vi "SendChargingCAN.vi"(8 "error in (no error)":errorcluster, 11 "interface object in":refnum<k20>) -> (0 "error out":errorcluster, 3 "interface object out":refnum<k20>)   [LabVIEW 2014]
uses:
  <vilib>/RioEmbeddedCAN/RioEmbeddedCAN.llb/CANFrameControl.ctl
  <vilib>/RioEmbeddedCAN/RioEmbeddedCAN.llb/CANWaitTransmitComplete.vi
  Global Data.vi
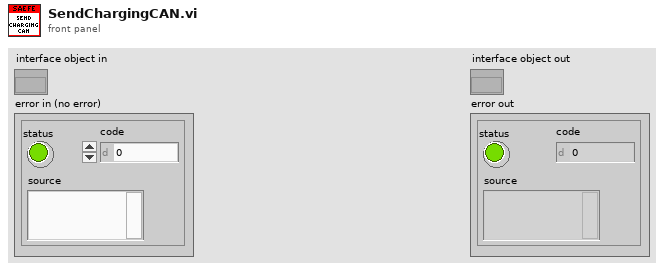
[diagram p1: front panel]
types:
  T1 = typedef "CANFrameControl.ctl" = cluster{"identifier":u32, "extended?":bool, "type":u8, "payload":u8[]}
  T2 = typedef "BMS Telemetry.ctl" = cluster{"bBMSIgnition":bool, "bBMSChargerMains":bool, "bBMSFastCharge":bool, "bBMSChargerEnabled":bool, "eBMSCarState":enum16{"Off", "On, Not Charging", "Charging", "Charging Finished", "Charging Error"}, "eBMSChargingState":enum16{"Disconnected", "Pre-charging", "Main Charging", "Balancing", "Charging Finished OK", "Charging Error"}, "tBMSChargeStage":u16, "eBMSLastChargeError":enum16{"No Error", "No Cell Communication", "No Cell Communication - Non CAN Charger", "Maximum charging stage duration expired", "Cell Communication Lost during Charge", "Cannot set balancing voltage", "Cell temps too high", "No Comms so can't determine temp", "# of Cells Mismatch", "Cells Overvoltage", "Cell Protection Event occured."}, "NBMSNumCells":u8, "bBMSUnderVProtection":bool, "bBMSOverVProtection":bool, "bBMSOverTProtection":bool, "bBMSLeakageProtection":bool, "bBMSNoCellCommsError":bool, "bBMSLowVReduction":bool, "bBMSHighTReduction":bool, "VCellMin":dbl, "VCellMax":dbl, "VCellMean":dbl, "VTotal":dbl, "TCellMin":dbl, "TCellMax":dbl, "TCellMean":dbl, "VCells":cluster{"[51]":dbl, "[52]":dbl, "[53]":dbl, "[54]":dbl, "[55]":dbl, "[56]":dbl, "[57]":dbl, "[58]":dbl, "[59]":dbl, "[60]":dbl, "[61]":dbl, "[62]":dbl, "[63]":dbl, "[64]":dbl, "[65]":dbl, "[66]":dbl, "[67]":dbl, "[34]":dbl, "[35]":dbl, "[36]":dbl, "[37]":dbl, "[38]":dbl, "[39]":dbl, "[40]":dbl, "[41]":dbl, "[42]":dbl, "[43]":dbl, "[44]":dbl, "[45]":dbl, "[46]":dbl, "[47]":dbl, "[48]":dbl, "[49]":dbl, "[50]":dbl, "[17]":dbl, "[18]":dbl, "[19]":dbl, "[20]":dbl, "[21]":dbl, "[22]":dbl, "[23]":dbl, "[24]":dbl, "[25]":dbl, "[26]":dbl, "[27]":dbl, "[28]":dbl, "[29]":dbl, "[30]":dbl, "[31]":dbl, "[32]":dbl, "[33]":dbl, "[0]":dbl, "[1]":dbl, "[2]":dbl, "[3]":dbl, "[4]":dbl, "[5]":dbl, "[6]":dbl, "[7]":dbl, "[8]":dbl, "[9]":dbl, "[10]":dbl, "[11]":dbl, "[12]":dbl, "[13]":dbl, "[14]":dbl, "[15]":dbl, "[16]":dbl}, "TCells":cluster{"[55]":dbl, "[56]":dbl, "[57]":dbl, "[58]":dbl, "[59]":dbl, "[60]":dbl, "[61]":dbl, "[62]":dbl, "[63]":dbl, "[64]":dbl, "[65]":dbl, "[66]":dbl, "[67]":dbl, "[68]":dbl, "[69]":dbl, "[70]":dbl, "[17]":dbl, "[38]":dbl, "[39]":dbl, "[40]":dbl, "[41]":dbl, "[42]":dbl, "[43]":dbl, "[44]":dbl, "[45]":dbl, "[46]":dbl, "[47]":dbl, "[48]":dbl, "[49]":dbl, "[50]":dbl, "[51]":dbl, "[52]":dbl, "[53]":dbl, "[54]":dbl, "[21]":dbl, "[22]":dbl, "[23]":dbl, "[24]":dbl, "[25]":dbl, "[26]":dbl, "[27]":dbl, "[28]":dbl, "[29]":dbl, "[30]":dbl, "[31]":dbl, "[32]":dbl, "[33]":dbl, "[34]":dbl, "[35]":dbl, "[36]":dbl, "[37]":dbl, "[0]":dbl, "[1]":dbl, "[2]":dbl, "[3]":dbl, "[4]":dbl, "[5]":dbl, "[6]":dbl, "[7]":dbl, "[8]":dbl, "[9]":dbl, "[10]":dbl, "[11]":dbl, "[12]":dbl, "[13]":dbl, "[14]":dbl, "[15]":dbl, "[16]":dbl}, "bChargerConnected":bool, "VChargerSetpoint":dbl, "IChargerSetpoint":dbl, "VChargerActual":dbl, "IChargerActual":dbl, "BCells":cluster{"[51]":dbl, "[52]":dbl, "[53]":dbl, "[54]":dbl, "[55]":dbl, "[56]":dbl, "[57]":dbl, "[58]":dbl, "[59]":dbl, "[60]":dbl, "[61]":dbl, "[62]":dbl, "[63]":dbl, "[64]":dbl, "[65]":dbl, "[66]":dbl, "[67]":dbl, "[34]":dbl, "[35]":dbl, "[36]":dbl, "[37]":dbl, "[38]":dbl, "[39]":dbl, "[40]":dbl, "[41]":dbl, "[42]":dbl, "[43]":dbl, "[44]":dbl, "[45]":dbl, "[46]":dbl, "[47]":dbl, "[48]":dbl, "[49]":dbl, "[50]":dbl, "[17]":dbl, "[18]":dbl, "[19]":dbl, "[20]":dbl, "[21]":dbl, "[22]":dbl, "[23]":dbl, "[24]":dbl, "[25]":dbl, "[26]":dbl, "[27]":dbl, "[28]":dbl, "[29]":dbl, "[30]":dbl, "[31]":dbl, "[32]":dbl, "[33]":dbl, "[0]":dbl, "[1]":dbl, "[2]":dbl, "[3]":dbl, "[4]":dbl, "[5]":dbl, "[6]":dbl, "[7]":dbl, "[8]":dbl, "[9]":dbl, "[10]":dbl, "[11]":dbl, "[12]":dbl, "[13]":dbl, "[14]":dbl, "[15]":dbl, "[16]":dbl}}
  T3 = enum16{"Disconnected", "Pre-charging", "Main Charging", "Balancing", "Charging Finished OK", "Charging Error"}
  T4 = enum16{"No Error", "No Cell Communication", "No Cell Communication - Non CAN Charger", "Maximum charging stage duration expired", "Cell Communication Lost during Charge", "Cannot set balancing voltage", "Cell temps too high", "No Comms so can't determine temp", "# of Cells Mismatch", "Cells Overvoltage", "Cell Protection Event occured."}
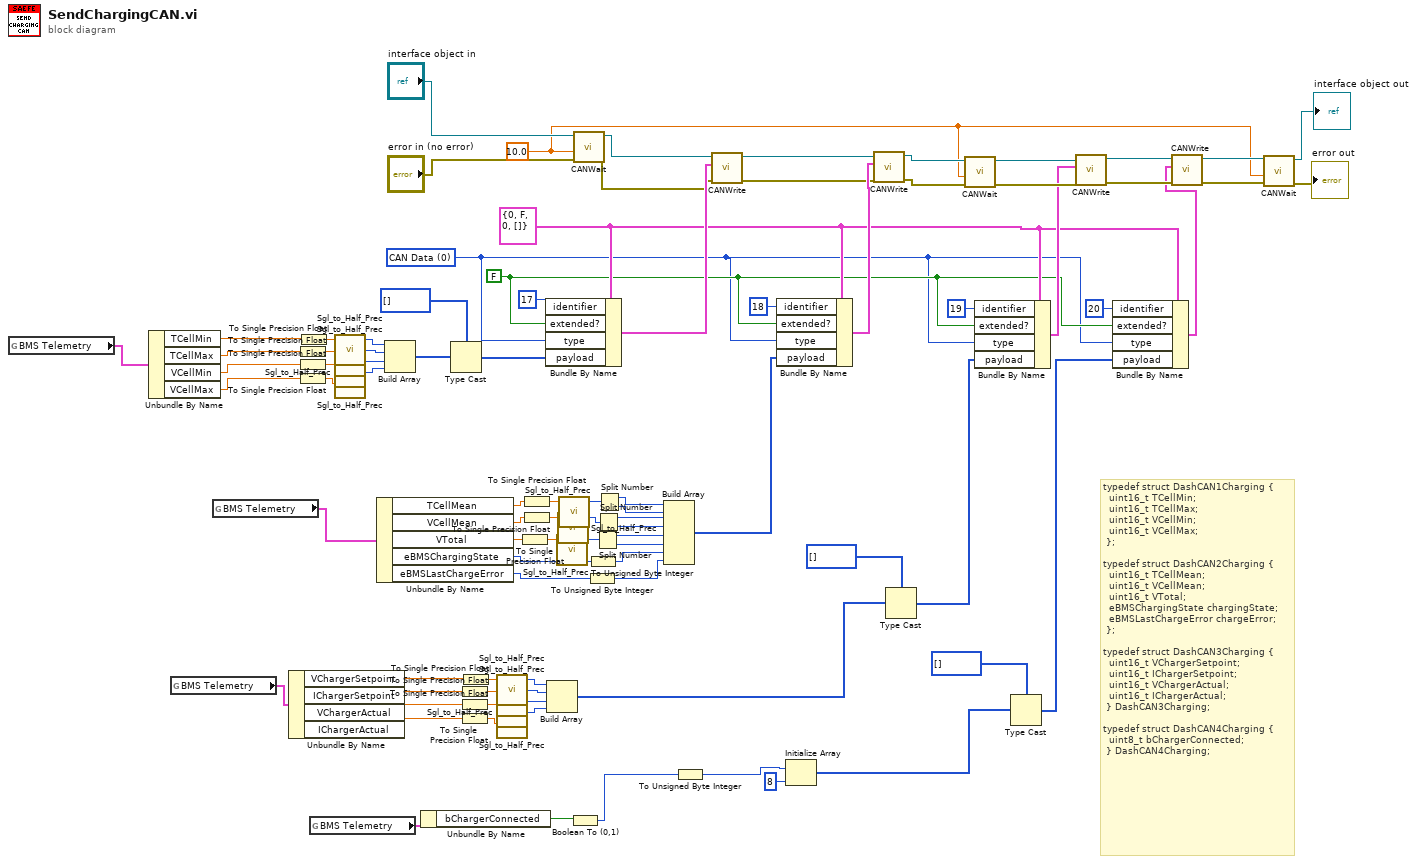
[diagram p0: block diagram]
diagram:
  w36 = 10.0 ("timeout (0 s)")
  w25 = u8 0 items=["CAN Data", "CAN Remote"] ("type")
  w27 = T1 {"identifier"=0, "extended?"=FALSE, "type"=0, "payload"=[]} ("CAN frame")
  w26 = FALSE ("extended?")
  # "typedef struct DashCAN1Charging {\n\t\tuint16_t TCellMin;\n\t\tuint16_t TCellMax;\n\t\tuint16_t VCellMin;\n\t\tuint16_t VCellMax;\n\t};\n\ntypedef struct DashCAN2Charging {\n\t\tuint16_t TCellMean;\n\t\tuint16_t VCellMean;\n\t\tuint16_t VTotal;\n\t\teBMSChargingState chargingState;\n\t\teBMSLastChargeError chargeError;\n\t};\n\ntypedef struct DashCAN3Charging {\n\t\tuint16_t VChargerSetpoint;\n\t\tuint16_t IChargerSetpoint;\n\t\tuint16_t VChargerActual;\n\t\tuint16_t IChargerActual;\n\t} DashCAN3Charging;\n\ntypedef struct DashCAN4Charging {\n\t\tuint8_t bChargerConnected;\n\t} DashCAN4Charging;"
  n1 = global read "Global Data.vi" "BMS Telemetry"() -> (w61:T2)
  n2 = Unbundle By Name(w61) -> ("TCellMin"=w60:dbl, "TCellMax"=w59:dbl, "VCellMin"=w58:dbl, "VCellMax"=w57:dbl)
  n3 = global read "Global Data.vi" "BMS Telemetry"() -> (w16:T2)
  n4 = global read "Global Data.vi" "BMS Telemetry"() -> (w54:T2)
  n5 = Unbundle By Name(w16) -> ("VChargerSetpoint"=w15:dbl, "IChargerSetpoint"=w14:dbl, "VChargerActual"=w13:dbl, "IChargerActual"=w12:dbl)
  n6 = To Single Precision Float(number=w59) -> (single precision float=w78:sgl)
  n7 = To Single Precision Float(number=w58) -> (single precision float=w76:sgl)
  n8 = To Single Precision Float(number=w57) -> (single precision float=w70:sgl)
  n9 = To Single Precision Float(number=w60) -> (single precision float=w77:sgl)
  n10 = global read "Global Data.vi" "BMS Telemetry"() -> (w7:T2)
  n11 = call "Sgl_to_Half_Prec.vi"("SGL"=w77) -> ("Half Precision Floating Point"=w82:u16)  [unwired: 4 in]
  n12 = call "Sgl_to_Half_Prec.vi"("SGL"=w78) -> ("Half Precision Floating Point"=w81:u16)  [unwired: 4 in]
  n13 = call "Sgl_to_Half_Prec.vi"("SGL"=w76) -> ("Half Precision Floating Point"=w80:u16)  [unwired: 4 in]
  n14 = call "Sgl_to_Half_Prec.vi"("SGL"=w70) -> ("Half Precision Floating Point"=w79:u16)  [unwired: 4 in]
  n15 = Unbundle By Name(w54) -> ("TCellMean"=w53:dbl, "VCellMean"=w52:dbl, "VTotal"=w51:dbl, "eBMSChargingState"=w50:T3, "eBMSLastChargeError"=w49:T4)
  n16 = Build Array(w82, w81, w80, w79) -> (w83:u16[])
  n17 = Unbundle By Name(w7) -> ("bChargerConnected"=w6:bool)
  n18 = Type Cast(type=u8[] [], x=w83) -> (*(type *) &x=w85:u8[])
  n19 = To Single Precision Float(number=w14) -> (single precision float=w20:sgl)
  n20 = To Single Precision Float(number=w13) -> (single precision float=w18:sgl)
  n21 = To Single Precision Float(number=w12) -> (single precision float=w17:sgl)
  n22 = To Single Precision Float(number=w15) -> (single precision float=w19:sgl)
  n23 = call "Sgl_to_Half_Prec.vi"("SGL"=w19) -> ("Half Precision Floating Point"=w24:u16)  [unwired: 4 in]
  n24 = call "Sgl_to_Half_Prec.vi"("SGL"=w20) -> ("Half Precision Floating Point"=w23:u16)  [unwired: 4 in]
  n25 = call "Sgl_to_Half_Prec.vi"("SGL"=w18) -> ("Half Precision Floating Point"=w22:u16)  [unwired: 4 in]
  n26 = call "Sgl_to_Half_Prec.vi"("SGL"=w17) -> ("Half Precision Floating Point"=w21:u16)  [unwired: 4 in]
  n27 = To Single Precision Float(number=w51) -> (single precision float=w56:sgl)
  n28 = To Single Precision Float(number=w53) -> (single precision float=w75:sgl)
  n29 = To Single Precision Float(number=w52) -> (single precision float=w74:sgl)
  n30 = Bundle By Name(cluster=w27, "identifier"=u32 17, "extended?"=w26, "type"=w25, "payload"=w85) -> (w88:T1)
  n31 = Build Array(w24, w23, w22, w21) -> (w11:u16[])
  n32 = call "Sgl_to_Half_Prec.vi"("SGL"=w56) -> ("Half Precision Floating Point"=w55:u16)  [unwired: 4 in]
  n33 = call "Sgl_to_Half_Prec.vi"("SGL"=w74) -> ("Half Precision Floating Point"=w73:u16)  [unwired: 4 in]
  n34 = call "Sgl_to_Half_Prec.vi"("SGL"=w75) -> ("Half Precision Floating Point"=w72:u16)  [unwired: 4 in]
  n35 = Boolean To (0,1)(Boolean=w6) -> (0, 1=w2:i16)
  n36 = call-poly <vilib>:"CANWait.vi"("error in (no error)"="error in (no error)", "timeout (0 s)"=w36, "interface object in"="interface object in") -> ("error out"=w66:errorcluster, "interface object out"=w67:refnum<k20>)  [unwired: 7 in]
  n37 = To Unsigned Byte Integer(number=w49) -> (unsigned 8bit integer=w41:u8)
  n38 = To Unsigned Byte Integer(number=w50) -> (unsigned 8bit integer=w42:u8)
  n39 = Split Number(x=w55) -> (hi(x)=w44:u8, lo(x)=w43:u8)
  n40 = Split Number(x=w73) -> (hi(x)=w46:u8, lo(x)=w45:u8)
  n41 = Split Number(x=w72) -> (hi(x)=w48:u8, lo(x)=w47:u8)
  n42 = Build Array(w48, w47, w46, w45, w44, w43, w42, w41) -> (w71:u8[])
  n43 = To Unsigned Byte Integer(number=w2) -> (unsigned 8bit integer=w1:u8)
  n44 = call <vilib>:"CANWrite.vi"("error in (no error)"=w66, "CAN frame"=w88, "interface object in"=w67) -> ("error out"=w62:errorcluster, "interface object out"=w63:refnum<k20>)  [unwired: 7 in]
  n45 = Bundle By Name(cluster=w27, "identifier"=u32 18, "extended?"=w26, "type"=w25, "payload"=w71) -> (w87:T1)
  n46 = Initialize Array(w1, 8 ("dimension size")) -> (w4:u8[])
  n47 = call <vilib>:"CANWrite.vi"("error in (no error)"=w62, "CAN frame"=w87, "interface object in"=w63) -> ("error out"=w64:errorcluster, "interface object out"=w65:refnum<k20>)  [unwired: 7 in]
  n48 = Type Cast(type=u8[] [], x=w11) -> (*(type *) &x=w9:u8[])
  n49 = call-poly <vilib>:"CANWait.vi"("error in (no error)"=w64, "timeout (0 s)"=w36, "interface object in"=w65) -> ("error out"=w34:errorcluster, "interface object out"=w35:refnum<k20>)  [unwired: 7 in]
  n50 = Bundle By Name(cluster=w27, "identifier"=u32 19, "extended?"=w26, "type"=w25, "payload"=w9) -> (w29:T1)
  n51 = Type Cast(type=u8[] [], x=w4) -> (*(type *) &x=w3:u8[])
  n52 = call <vilib>:"CANWrite.vi"("error in (no error)"=w34, "CAN frame"=w29, "interface object in"=w35) -> ("error out"=w32:errorcluster, "interface object out"=w33:refnum<k20>)  [unwired: 7 in]
  n53 = Bundle By Name(cluster=w27, "identifier"=u32 20, "extended?"=w26, "type"=w25, "payload"=w3) -> (w28:T1)
  n54 = call <vilib>:"CANWrite.vi"("error in (no error)"=w32, "CAN frame"=w28, "interface object in"=w33) -> ("error out"=w37:errorcluster, "interface object out"=w38:refnum<k20>)  [unwired: 7 in]
  n55 = call-poly <vilib>:"CANWait.vi"("error in (no error)"=w37, "timeout (0 s)"=w36, "interface object in"=w38) -> ("error out"=→"error out":errorcluster, "interface object out"=→"interface object out":refnum<k20>)  [unwired: 7 in]
